vi "looking at the data.vi"() -> ()   [LabVIEW 2020]
uses:
  <vilib>/measure/NI_MAPro.lvlib
  <vilib>/measure/maresamp.llb/Resample Waveform (single shot).vi
  file handler/VFH-file_cluster-Expensive.ctl
  file handler/VFH-VNA_File_Handler.lvlib
  file handler/VFH-file_cluster-LabVIEWVNA.ctl
  file handler/VFH-file_cluster-NanoVNA.ctl
  analyse freq.ctl
panel:
  out "first subarray 3":dbl[](array[numeric])
  out "size(s) 2":i32
  out "size(s)":i32
  out "x-y 2":dbl
  out "x-y":dbl
  out "Y":dbl[](array[numeric])
  out "appended array 2":i32[](array[numeric])
  out "appended array":dbl[](array[numeric])
  out "Array 6":i32[](array[numeric])
  out "first subarray 2":dbl[](array[numeric])
  out "second subarray":dbl[](array[numeric])
  out "first subarray":dbl[](array[numeric])
  out "Array 5":dbl[](array[numeric])
  out "Array 4":dbl[](array[numeric])
  out "Array 3":dbl[](array[numeric])
  out "Array 2":i32[](array[numeric])
  out "Array":dbl[][](array[numeric])
  out "Freq info ex":T1 {"resolution" format="%#_6p"; "Delta" format="%#_6p"; "Min" format="%#_6p"; "Max" format="%#_6p"}
  out "Freq info LV":T1 {"resolution" format="%#_6p"; "Delta" format="%#_6p"; "Min" format="%#_6p"; "Max" format="%#_6p"}
  out "Freq info NV":T1 {"resolution" format="%#_6p"; "Delta" format="%#_6p"; "Min" format="%#_6p"; "Max" format="%#_6p"}
  in  "Tab Control":T2(tab)
  out "avg output NV":T3
  out "avg output LV":T4
  out "output EX":T5
  out "Waveform Graph":dbl[][](graph)
  out "Waveform Graph 6":dbl[][](graph)
  out "Waveform Graph 7":waveform(dbl)[](graph)
  out "Waveform Graph 2":dbl[][](graph)
  out "Waveform Graph 4":waveform(dbl)[](graph)
  out "Waveform Graph 5":dbl[][](graph)
  out "Waveform Graph 3":dbl[][](graph)
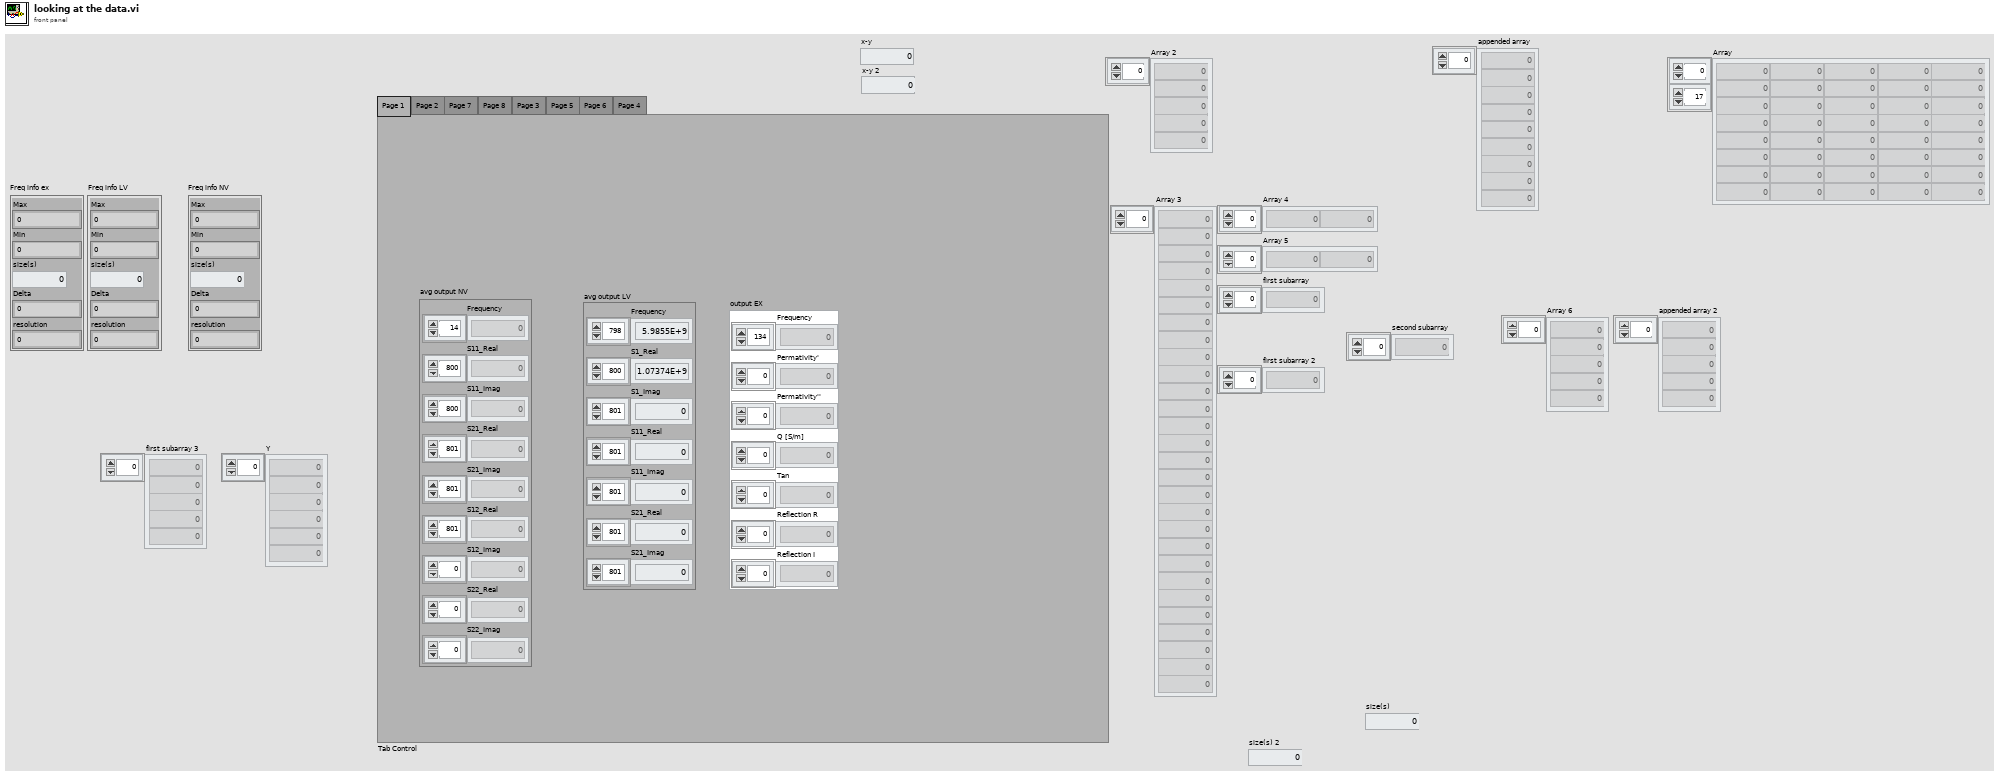
[diagram p1: front panel]
types:
  T1 = typedef "analyse freq.ctl" = cluster{"Max":dbl, "Min":dbl, "size(s)":i32, "Delta":dbl, "resolution":dbl}
  T2 = enum32{"Page 1", "Page 2", "Page 7", "Page 8", "Page 3", "Page 5", "Page 6", "Page 4"}
  T3 = typedef "VFH-VNA_File_Handler.lvlib/VFH-file_cluster-NanoVNA.ctl" = cluster{"Frequency":dbl[], "S11_Real":dbl[], "S11_Imag":dbl[], "S21_Real":dbl[], "S21_Imag":dbl[], "S12_Real":dbl[], "S12_Imag":dbl[], "S22_Real":dbl[], "S22_Imag":dbl[]}
  T4 = typedef "VFH-VNA_File_Handler.lvlib/VFH-file_cluster-LabVIEWVNA.ctl" = cluster{"Frequency":dbl[], "S1_Real":dbl[], "S1_Imag":dbl[], "S11_Real":dbl[], "S11_Imag":dbl[], "S21_Real":dbl[], "S21_Imag":dbl[]}
  T5 = typedef "VFH-VNA_File_Handler.lvlib/VFH-file_cluster-Expensive.ctl" = cluster{"Frequency":dbl[], "Permativity'":dbl[], "Permativity''":dbl[], "Q [S/m]":dbl[], "Tan":dbl[], "Reflection R":dbl[], "Reflection I":dbl[]}
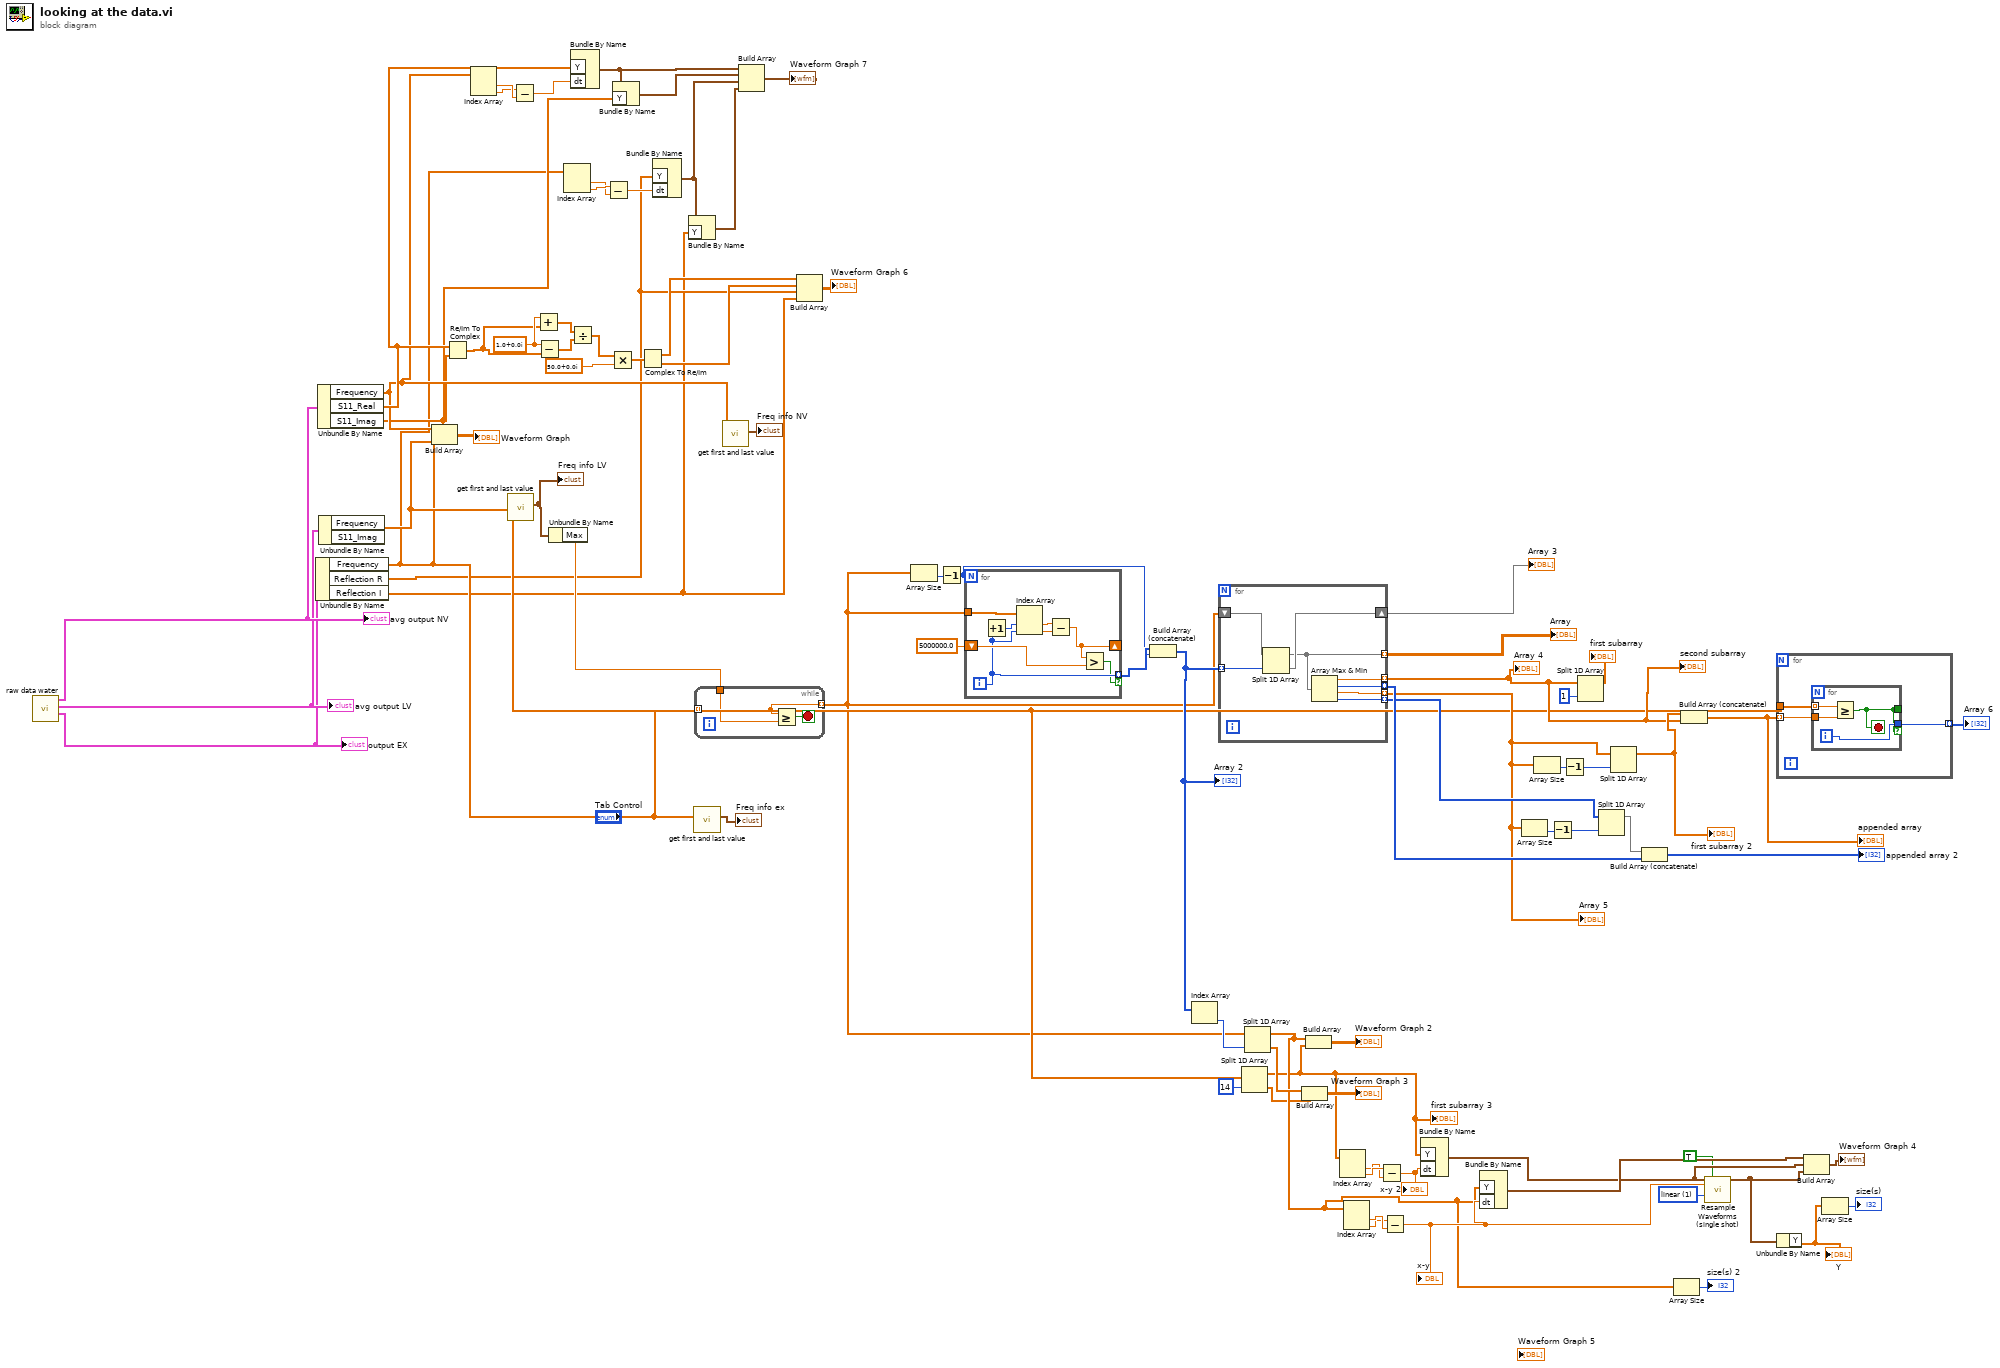
[diagram p0: block diagram]
diagram:
  w26 = cdb 1.0+0.0i ("x")
  w41 = u16 1 items=["coerce", "linear", "spline", "FIR filter"] ("interpolation mode")
  n1 = call "raw data water.vi"() -> ("output R140"=w80:T5, "avg output LV"=w81:T4, "avg output NV"=w82:T3)  [unwired: 9 in]
  "avg output NV" <- w82
  "avg output LV" <- w81
  "output EX" <- w80
  n2 = Unbundle By Name(w80) -> ("Frequency"=w7:dbl[], "Reflection R"=w5:dbl[], "Reflection I"=w4:dbl[])
  n3 = Unbundle By Name(w82) -> ("Frequency"=w16:dbl[], "S11_Real"=w17:dbl[], "S11_Imag"=w11:dbl[])
  n4 = Unbundle By Name(w81) -> ("Frequency"=w33:dbl[])  [unwired: 1 out]
  n5 = Build Array(w16, w33, w7) -> (→"Waveform Graph":dbl[][])
  n6 = Re/Im To Complex(1:w11, 2:w17) -> (0:w21:cdb[])
  n7 = Index Array(array=w16) -> (element #1=w15:dbl, element #2=w14:dbl)  [unwired: 2 in]
  n8 = call "get first and last value.vi"("Array"=w33) -> ("Freq info"=w75:T1)  [unwired: 10 in]
  "Freq info LV" <- w75
  n9 = Subtract(x=w14, y=w15) -> (x-y=w13:dbl)
  n10 = Add(x=w26, y=w21) -> (x+y=w25:cdb[])
  n11 = Subtract(x=w26, y=w21) -> (x-y=w24:cdb[])
  n12 = Unbundle By Name(w75) -> ("Max"=w76:dbl)
  n13 = Index Array(array=w7) -> (element #1=w8:dbl, element #2=w9:dbl)  [unwired: 2 in]
  n14 = Divide(x=w25, y=w24) -> (x/y=w23:cdb[])
  n15 = Bundle By Name("Y"=w17, "dt"=w13) -> (w12:waveform(dbl))  [unwired: 1 in]
  n16 = Subtract(x=w9, y=w8) -> (x-y=w6:dbl)
  n17 = Multiply(x=w23, y=cdb 50.0+0.0i) -> (x*y=w20:cdb[])
  n18 = Bundle By Name(cluster=w12, "Y"=w11) -> (w10:waveform(dbl))
  n19 = Complex To Re/Im(x + iy=w20) -> (x=w19:dbl[], y=w18:dbl[])
  n20 = Bundle By Name("Y"=w5, "dt"=w6) -> (w3:waveform(dbl))  [unwired: 1 in]
  n21 = Bundle By Name(cluster=w3, "Y"=w4) -> (w2:waveform(dbl))
  n22 = call "get first and last value.vi"("Array"=w7) -> ("Freq info"=→"Freq info ex":T1)  [unwired: 10 in]
  n23 = while {
    tunnel: w7 -> [w83] mode=indexing
    tunnel: w76 -> [w85]
    tunnel: [w83] -> w30 mode=indexing
    stop <- w84 stop-if-true
    n24 = Greater Or Equal?(x=w83, y=w85) -> (x >= y?=w84:bool)
  }
  n25 = call "get first and last value.vi"("Array"=w16) -> ("Freq info"=→"Freq info NV":T1)  [unwired: 10 in]
  n26 = Build Array(w12, w10, w3, w2) -> (→"Waveform Graph 7":waveform(dbl)[])
  n27 = Build Array(w19, w18, w5, w4) -> (→"Waveform Graph 6":dbl[][])
  n28 = Array Size(array=w30) -> (size(s)=w73:i32)
  n29 = Decrement(x=w73) -> (x-1=w69:i32)
  n30 = for {
    N: w69 -> [_]
    tunnel: w30 -> [w93]
    shift-right: [w89] -> _
    shift-left: 5000000.0 -> [w88]
    tunnel: [w87] -> w70 mode=indexing if=w86
    i -> [w87]
    n31 = Increment(x=w87) -> (x+1=w92:i32)
    n32 = Index Array(array=w93, index #1=w92, index #2=w87) -> (element #1=w91:dbl, element #2=w90:dbl)
    n33 = Subtract(x=w91, y=w90) -> (x-y=w89:dbl)
    n34 = Greater?(x=w89, y=w88) -> (0:w86:bool)
  }
  n35 = Build Array (concatenate)(w70, w69) -> (w53:i32[])
  "Array 2" <- w53
  n36 = Index Array(array=w53) -> (element=w52:i32)  [unwired: 1 in]
  n37 = for {
    shift-right: [w100] -> w71
    shift-left: w30 -> [w101]
    tunnel: [w98] -> w74 mode=indexing
    tunnel: w53 -> [w99] mode=indexing
    tunnel: [w97] -> w61 mode=indexing
    tunnel: [w96] -> w56 mode=indexing
    tunnel: [w95] -> w60 mode=indexing
    tunnel: [w94] -> w57 mode=indexing
    n38 = Split 1D Array(array=w101, index=w99) -> (first subarray=w98:dbl[], second subarray=w100:dbl[])
    n39 = Array Max & Min(array=w98) -> (max value=w97:dbl, max index (indices)=w95:i32, min value=w96:dbl, min index (indices)=w94:i32)
  }
  "Array" <- w74
  "Array 3" <- w71
  "Array 4" <- w61
  "Array 5" <- w56
  "second subarray" <- w61
  n40 = Split 1D Array(array=w33, index=14) -> (first subarray=w29:dbl[], second subarray=w31:dbl[])
  "first subarray 3" <- w29
  n41 = Split 1D Array(array=w30, index=w52) -> (first subarray=w32:dbl[], second subarray=w49:dbl[])
  n42 = Build Array(w49, w31) -> (→"Waveform Graph 3":dbl[][])
  n43 = Build Array(w32, w29) -> (→"Waveform Graph 2":dbl[][])
  n44 = Index Array(array=w29) -> (element #1=w46:dbl, element #2=w47:dbl)  [unwired: 2 in]
  n45 = Index Array(array=w32) -> (element #1=w44:dbl, element #2=w43:dbl)  [unwired: 2 in]
  n46 = Subtract(x=w47, y=w46) -> (x-y=w45:dbl)
  "x-y 2" <- w45
  n47 = Subtract(x=w43, y=w44) -> (x-y=w40:dbl)
  "x-y" <- w40
  n48 = Bundle By Name("Y"=w29, "dt"=w45) -> (w38:waveform(dbl))  [unwired: 1 in]
  n49 = Bundle By Name("Y"=w32, "dt"=w40) -> (w39:waveform(dbl))  [unwired: 1 in]
  n50 = Array Size(array=w56) -> (size(s)=w58:i32)
  n51 = Array Size(array=w56) -> (size(s)=w66:i32)
  n52 = Decrement(x=w58) -> (x-1=w59:i32)
  n53 = Decrement(x=w66) -> (x-1=w65:i32)
  n54 = Split 1D Array(array=w61, index=1) -> (first subarray=→"first subarray":dbl[])  [unwired: 1 out]
  n55 = Split 1D Array(array=w57, index=w59) -> (first subarray=w55:i32[])  [unwired: 1 out]
  n56 = Split 1D Array(array=w56, index=w65) -> (first subarray=w64:dbl[])  [unwired: 1 out]
  "first subarray 2" <- w64
  n57 = Build Array (concatenate)(w55, w60) -> (→"appended array 2":i32[])
  n58 = Array Size(array=w32) -> (size(s)=→"size(s) 2":i32)
  n59 = Build Array (concatenate)(w64, w61) -> (w63:dbl[])
  "appended array" <- w63
  n60 = call-poly <vilib>:"Resample Waveforms (single shot).vi"("waveform in"=w38, "open interval? (F)"=TRUE, "dt"=w40, "interpolation mode"=w41) -> ("resampled waveform out"=w34:waveform(dbl))  [unwired: 8 in, 3 out]
  n61 = for {
    tunnel: w63 -> [w104] mode=indexing
    tunnel: w33 -> [w103]
    tunnel: [w102] -> w62 mode=indexing
    n62 = for {
      tunnel: w104 -> [w108]
      tunnel: w103 -> [w107] mode=indexing
      tunnel: [w105] -> _
      tunnel: [w106] -> w102 if=w105
      i -> [w106]
      stop <- w105 stop-if-true
      n63 = Greater Or Equal?(x=w107, y=w108) -> (x >= y?=w105:bool)
    }
  }
  "Array 6" <- w62
  n64 = Unbundle By Name(w34) -> ("Y"=w37:dbl[])
  "Y" <- w37
  n65 = Build Array(w39, w38, w34) -> (→"Waveform Graph 4":waveform(dbl)[])
  n66 = Array Size(array=w37) -> (size(s)=→"size(s)":i32)
